vi "ad discrete in.vi"(7 "data":u32, 8 "error in (no error)":errorcluster, 9 "range":i32, 10 "cha":i32, 11 "adh":i32) -> (0 "error out":errorcluster, 3 "function return":i32, 5 "data out":u32)   [LabVIEW 2021, in "libad4.lvlib"]
doc: "LIBAD4 function: ad_discrete_in (int32_t adh, int32_t cha, int32_t range, uint32_t *data);\n\nAllows a discrete value to be read from the DAQ. This value can be converted to a voltage representation via `ad_sample_to_float`.\nNote: the channel numbers must be constructed as follows `AD_CHA_TYPE_ANALOG_IN | 0x0001`, where `|` is the bitwise OR operation. The full list of prefixes are shown here: \n\nAD_CHA_TYPE_ANALOG_IN 0x01000000\nAD_CHA_TYPE_ANALOG_OUT 0x02000000\nAD_CHA_TYPE_DIGITAL_IO 0x03000000\nAD_CHA_TYPE_SYNC 0x05000000\nAD_CHA_TYPE_ROUTE 0x06000000\nAD_CHA_TYPE_CAN 0x07000000\nAD_CHA_TYPE_COUNTER 0x08000000\nAD_CHA_TYPE_ANALOG_COUNTER 0x09000000\n\nNote: 'cha constructor.vi' can be used to help calculate these values within labview."
uses:
  <userlib>/libad4/libad4.lvlib
  <userlib>/libad4/libad4.dll
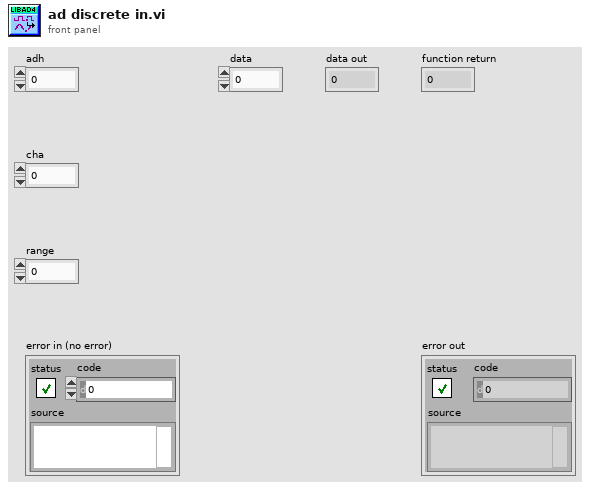
[diagram p1: front panel]
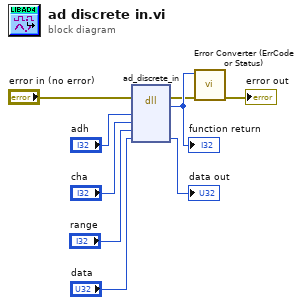
[diagram p0: block diagram]
diagram:
  n1 = dll-call lib="C:/Program Files/National Instruments/LabVIEW 2021/user.lib/libad4/libad4.*" fn="ad_discrete_in"(error in="error in (no error)", "adh"="adh", "cha"="cha", "range"="range", "data"="data") -> (error out=w2:errorcluster, "return type"=w9:i32, "data"=→"data out":u32)  [unwired: 5 in, 1 out]
  "function return" <- w9
  n2 = call <userlib>:"Error Converter (ErrCode or Status).vi"("error in (no error)"=w2, "error code"=w9) -> ("error out"=→"error out":errorcluster)  [unwired: 9 in]
